vi "FTW-ActorTemplate.vi"(0 "FTW Actor Instance Configuration":string="{\n  \"Identity\": \"ActorName\",\n  \"InboxAddress\": \"inproc://*\",\n  \"LoggerAddress\": \"\",\n  \"DebugEnableInboxLogging\": false,\n  \"DebugEnableJobLogging\": false,\n  \"LauncherAddress\": \"\"\n}", 11 "ErrorIn":errorcluster) -> (15 "Error":errorcluster)   [LabVIEW 2013]
uses:
  source/actor/Instance/FTW-ActorInstance.lvclass
  source/actor/Message/Base/FTW-Message.lvclass
  source/actor/Instance/FTW-ActorInstance.lvclass/FTW-ActorInstance.ctl
  source/actor/JobSequencer/FTW-SEQ-Current.vi
  source/actor/Message/Request/FTW-Message-IncomingRequest.lvclass
panel:
  # "Inputs"
  # "Outputs"
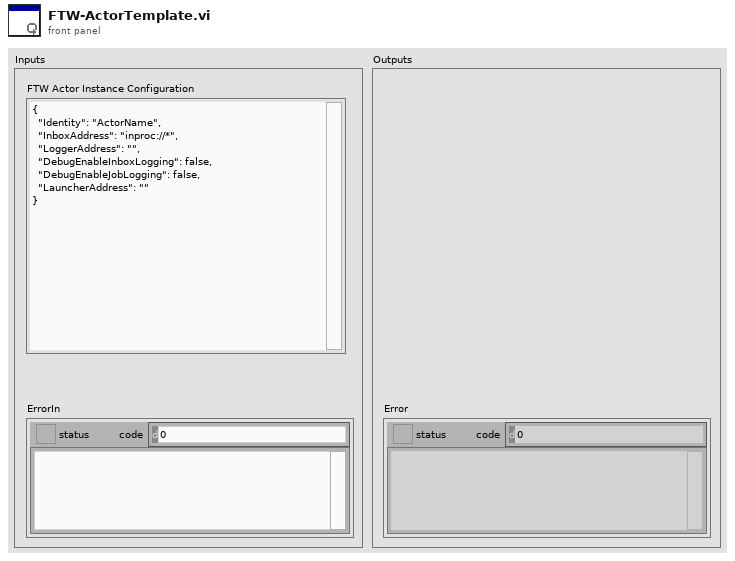
[diagram p1: front panel]
types:
  T1 = cluster{"Incoming Requests":refnum<event-registration>, "Local Messages":refnum<event-registration>, "Additional Registration Types":refnum<event-registration>}
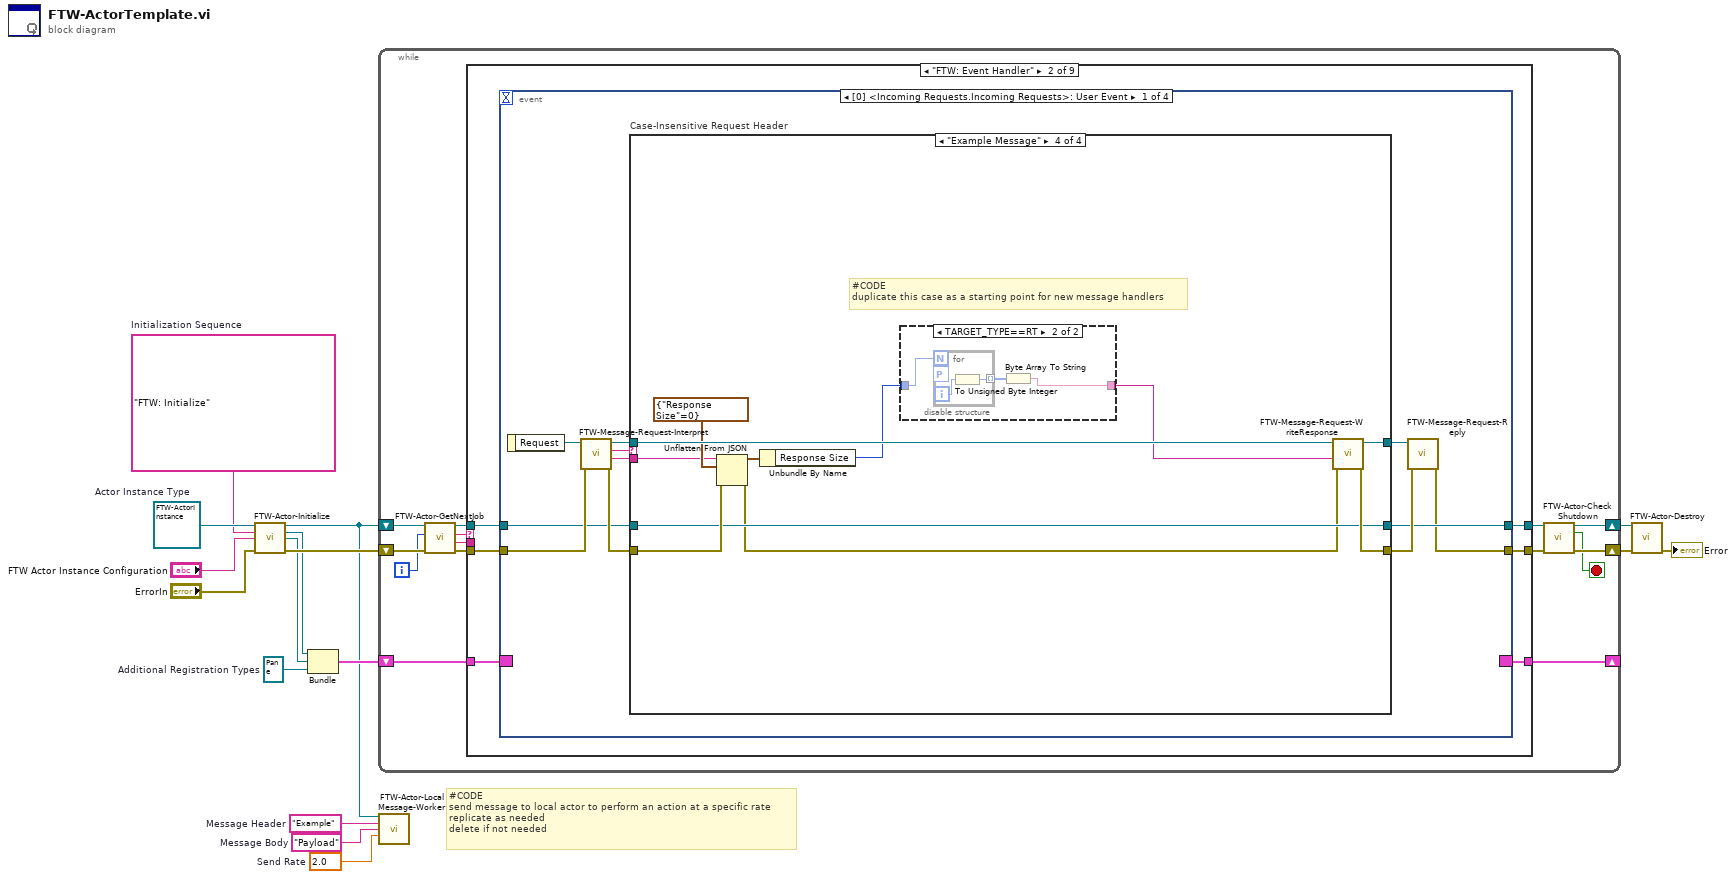
[diagram p0: block diagram]
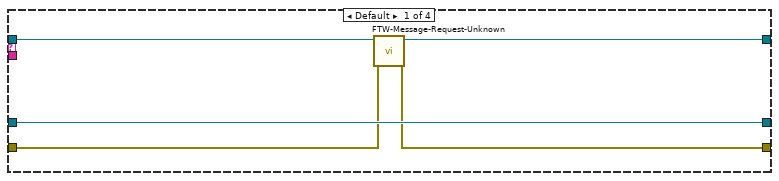
[diagram p3: hidden frame]
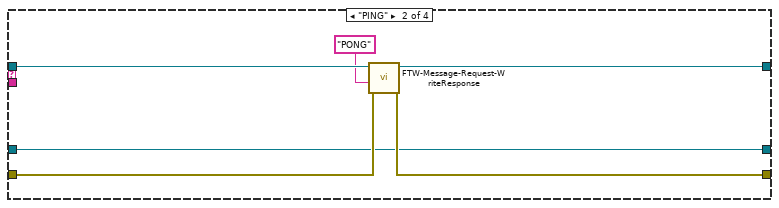
[diagram p4: hidden frame]
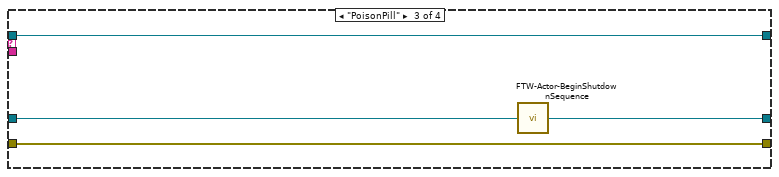
[diagram p5: hidden frame]
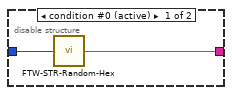
[diagram p6: hidden frame]
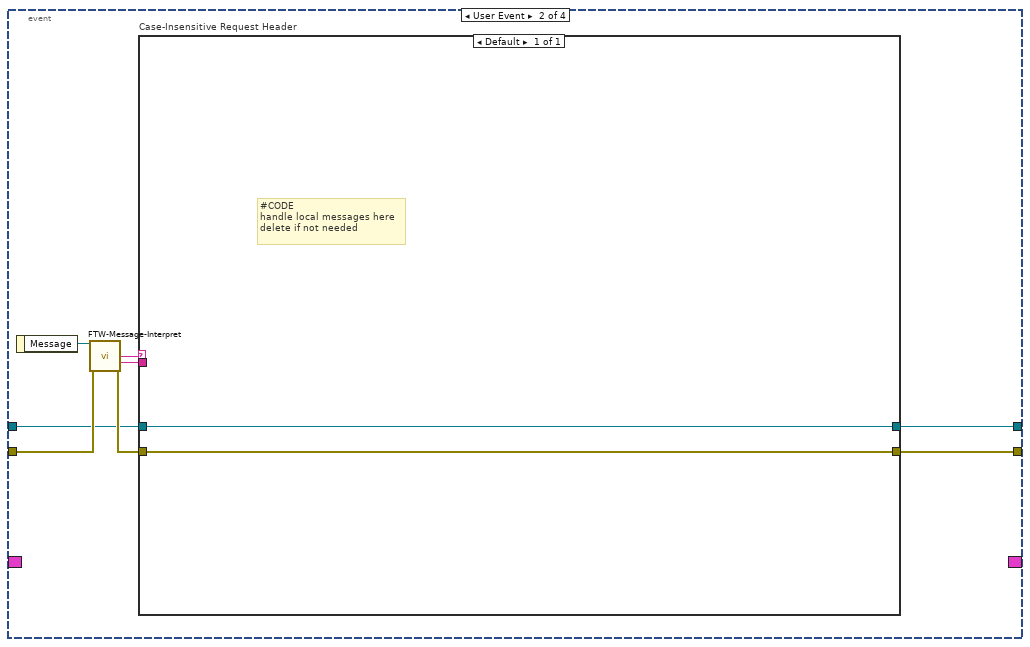
[diagram p7: hidden frame]
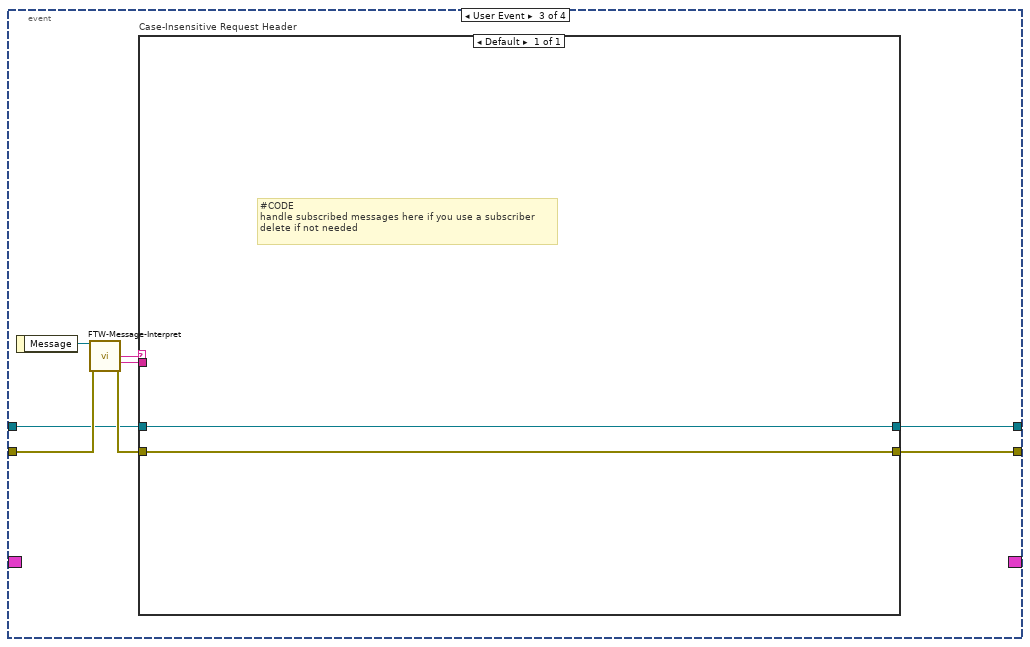
[diagram p8: hidden frame]
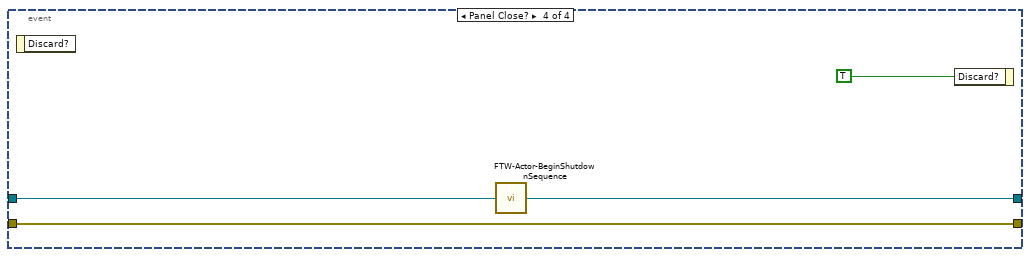
[diagram p9: hidden frame]
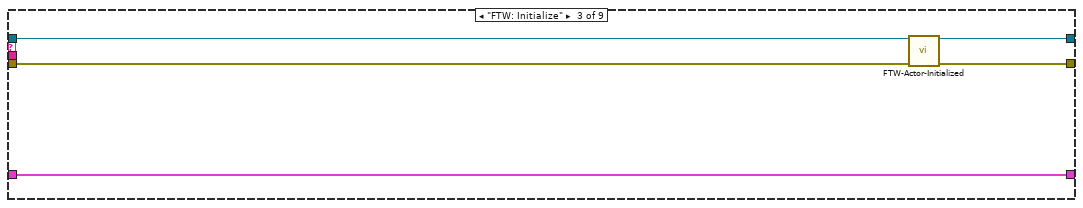
[diagram p10: hidden frame]
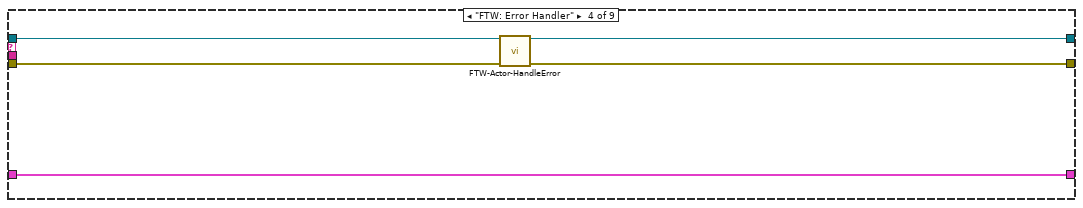
[diagram p11: hidden frame]
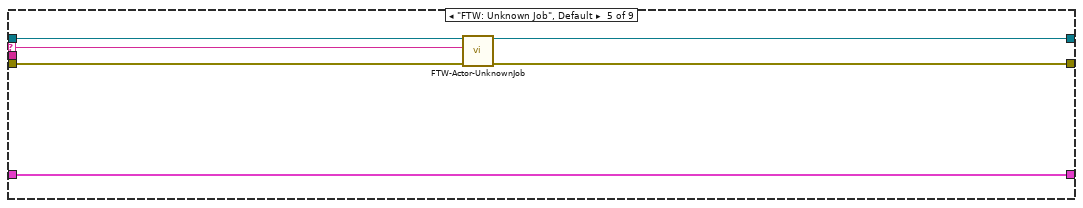
[diagram p12: hidden frame]
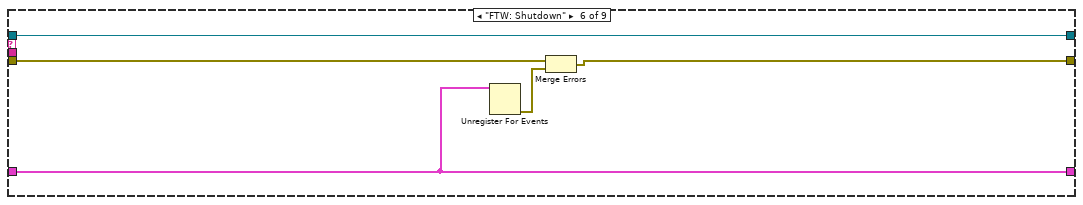
[diagram p13: hidden frame]
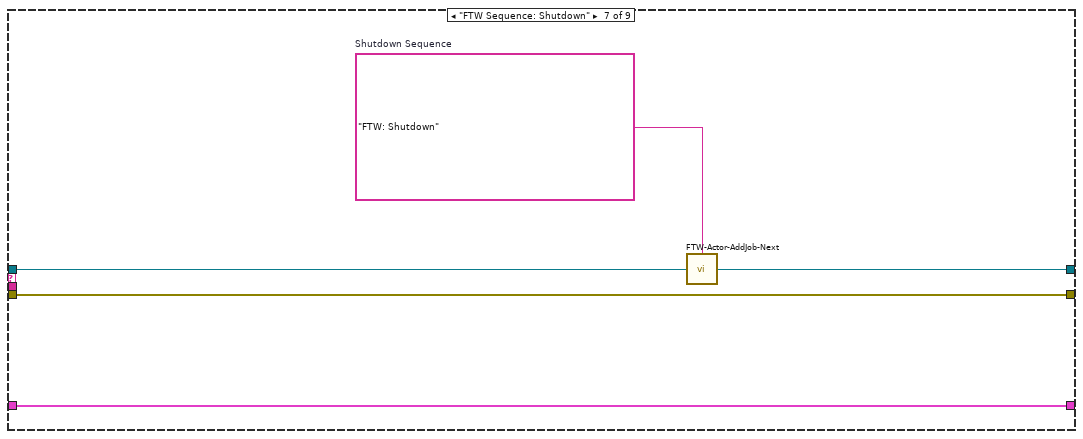
[diagram p14: hidden frame]
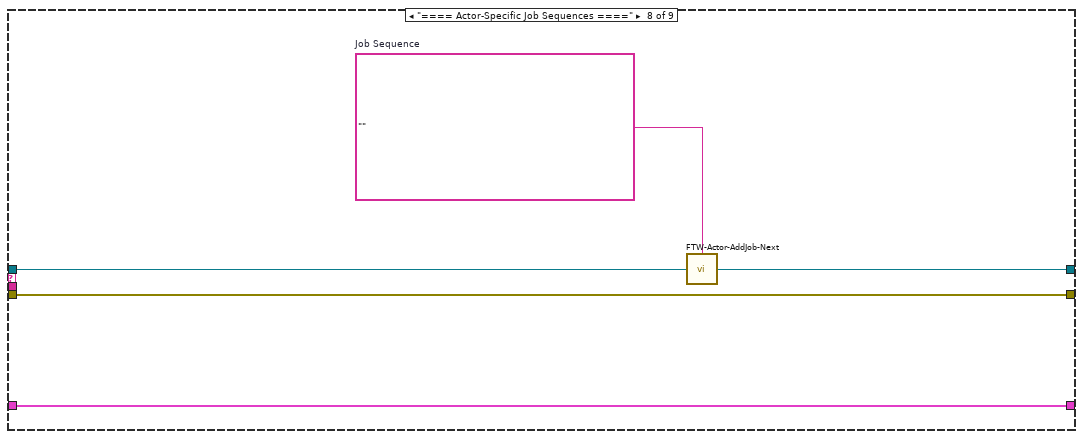
[diagram p15: hidden frame]
diagram:
  w1 = 2.0  # Send Rate
  w2 = "Payload"  # Message Body
  w3 = "Example"  # Message Header
  w5 = refnum<event-registration> refnum  # Additional Registration Types
  w12 = refnum<class "FTW-ActorInstance.lvclass"> refnum  # Actor Instance Type
  w11 = "FTW: Initialize"  # Initialization Sequence
  # "#CODE\nsend message to local actor to perform an action at a specific rate\nreplicate as needed\ndelete if not needed"
  n1 = call-dynamic "FTW-Actor-Initialize.vi"("FTW Actor Instance Type"=w12, "Initialization Job Sequence"=w11, "Actor Instance Configuration"="FTW Actor Instance Configuration", "error in"="ErrorIn") -> ("FTW Actor Instance"=w4:refnum<class "FTW-ActorInstance.lvclass">, "Incoming Requests"=w7:refnum<event-registration>, "Local Messages"=w6:refnum<event-registration>, "error out"=w13:errorcluster)  [unwired: 8 in]
  n2 = Bundle("Incoming Requests"=w7, "Local Messages"=w6, "Additional Registration Types"=w5) -> (w9:T1)  [unwired: 1 in]
  n3 = while {
    shift-right: [w20] -> w15
    shift-left: w13 -> [w27]
    shift-right: [w17] -> _
    shift-left: w9 -> [w30]
    shift-right: [w22] -> w16
    shift-left: w4 -> [w29]
    i -> [w18]
    stop <- w19 stop-if-true
    n4 = call "FTW-Actor-GetNextJob.vi"("error in"=w27, "Jobs Performed"=w18, "FTW Actor Instance"=w29) -> ("error out"=w26:errorcluster, "Job Data"=w24:string, "Job Name"=w25:string, "FTW Actor Instance out"=w28:refnum<class "FTW-ActorInstance.lvclass">)  [unwired: 5 in]
    n5 = case shown="\"FTW: Event Handler\"" w25 {
      selector: w25 -> [_ _ _ _ w118 _ _ _ _]
      tunnel: [w32 w39 w108 w113 w121 w127 w132 w137 w141] -> w21
      tunnel: w26 -> [w32 w38 w111 w115 w122 w128 w132 w137 w141]
      tunnel: w30 -> [w33 w34 w112 w117 w123 w124 w133 w138 w140]
      tunnel: [w33 w37 w112 w117 w123 w124 w133 w138 w140] -> w17
      tunnel: w24 -> [_ _ _ _ _ _ _ _ _]
      tunnel: [w31 w36 w109 w114 w119 w125 w130 w135 w139] -> w23
      tunnel: w28 -> [w31 w35 w110 w116 w120 w125 w131 w136 w139]
      frame "==== Featherweight Framework Jobs ====" {
      }
      frame "FTW: Event Handler" {
        n6 = event shown="[0] <Incoming Requests.Incoming Requests>: User Event" {
          selector: w34 -> [_ _ _ _]
          dyn-events: [_ _ _ _] -> w37
          timeout: _ -> [_ _ _ _]
          tunnel: [w42 w88 w98 w106] -> w39
          tunnel: w38 -> [w48 w89 w99 w106]
          tunnel: [w46 w87 w97 w104] -> w36
          tunnel: w35 -> [w45 w86 w96 w105]
          event User Event {
            n7 = event-data() -> ("Request"=w49:refnum<class "FTW-Message-IncomingRequest.lvclass">)  [unwired: 1 in]
            n8 = call "FTW-Message-Request-Interpret.vi"("error in"=w48, "FTW Incoming Request"=w49) -> ("error out"=w50:errorcluster, "Request Body"=w40:string, "Request Header"=w44:string, "FTW Incoming Request out"=w43:refnum<class "FTW-Message-IncomingRequest.lvclass">)  [unwired: 5 in, 1 out]
            n9 = case "Case-Insensitive Request Header" shown="\"Example Message\"" w44 {
              tunnel: [w53 w59 w64 w75] -> w47
              tunnel: w50 -> [w54 w60 w64 w76]
              tunnel: [w55 w58 w65 w72] -> w46
              tunnel: w45 -> [w55 w58 w63 w72]
              tunnel: w43 -> [w52 w61 w62 w74]
              tunnel: [w51 w57 w62 w73] -> w41
              tunnel: w40 -> [_ _ _ w66]
              frame Default {
                n10 = call "FTW-Message-Request-Unknown.vi"("error in"=w54, "FTW Incoming Request"=w52) -> ("error out"=w53:errorcluster, "FTW Incoming Request Out"=w51:refnum<class "FTW-Message-IncomingRequest.lvclass">)  [unwired: 8 in]
              }
              frame "PING" {
                n11 = call "FTW-Message-Request-WriteResponse.vi"("error in"=w60, "Response Body"="PONG" ("Response Header"), "FTW Incoming Request"=w61) -> ("error out"=w59:errorcluster, "FTW Incoming Request out"=w57:refnum<class "FTW-Message-IncomingRequest.lvclass">)  [unwired: 7 in]
              }
              frame "PoisonPill" {
                n12 = call "FTW-Actor-BeginShutdownSequence.vi"("FTW Actor Instance"=w63) -> ("FTW Actor Instance out"=w65:refnum<class "FTW-ActorInstance.lvclass">)  [unwired: 3 in]
              }
              frame "Example Message" {
                # "#CODE\nduplicate this case as a starting point for new message handlers"
                n13 = Unflatten From JSON(JSON string=w66, type and defaults=cluster{"Response Size":i32} {"Response Size"=0}, error in (no error)=w76) -> (value=w69:cluster{"Response Size":i32}, error out=w71:errorcluster)  [unwired: 4 in]
                n14 = Unbundle By Name(w69) -> ("Response Size"=w68:i32)
                n15 = disable-structure shown="TARGET_TYPE==RT" {
                  disable-tunnel: w68 -> [w78 w81]
                  disable-tunnel: [w77 w79] -> w67
                  frame condition #0 (active) {
                    n16 = call "FTW-STR-Random-Hex.vi"("String Length"=w78) -> ("Random Hex String"=w77:string)  [unwired: 3 in]
                  }
                  frame condition #1 {
                    n17 = for {
                      N: w81 -> [_]
                      workers-P: _ -> [_]
                      tunnel: [w82] -> w80 mode=indexing
                      i -> [w83]
                      n18 = To Unsigned Byte Integer(number=w83) -> (unsigned 8bit integer=w82:u8)
                    }
                    n19 = Byte Array To String(unsigned byte array=w80) -> (string=w79:string)
                  }
                }
                n20 = call "FTW-Message-Request-WriteResponse.vi"("error in"=w71, "Response Body"=w67, "FTW Incoming Request"=w74) -> ("error out"=w75:errorcluster, "FTW Incoming Request out"=w73:refnum<class "FTW-Message-IncomingRequest.lvclass">)  [unwired: 7 in]
              }
            }
            n21 = call "FTW-Message-Request-Reply.vi"("FTW: Reply Error"=w47, "FTW Incoming Request"=w41) -> ("error out"=w42:errorcluster)  [unwired: 8 in, 1 out]
          }
          event User Event {
            n22 = event-data() -> ("Message"=w90:refnum<class "FTW-Message.lvclass">)  [unwired: 1 in]
            n23 = call-dynamic "FTW-Message-Interpret.vi"("FTW Message"=w90, "error in"=w89) -> ("Message Header"=w84:string, "Message Body"=w85:string, "error out"=w91:errorcluster)  [unwired: 9 in, 2 out]
            n24 = case "Case-Insensitive Request Header" shown="Default" w84 {
              tunnel: [w92] -> w88
              tunnel: w91 -> [w92]
              tunnel: [w93] -> w87
              tunnel: w86 -> [w93]
              tunnel: w85 -> [_]
              frame Default {
                # "#CODE\nhandle local messages here\ndelete if not needed"
              }
            }
          }
          event User Event {
            n25 = event-data() -> ("Message"=w100:refnum<class "FTW-Message.lvclass">)  [unwired: 1 in]
            n26 = call-dynamic "FTW-Message-Interpret.vi"("FTW Message"=w100, "error in"=w99) -> ("Message Header"=w94:string, "Message Body"=w95:string, "error out"=w101:errorcluster)  [unwired: 9 in, 2 out]
            n27 = case "Case-Insensitive Request Header" shown="Default" w94 {
              tunnel: [w102] -> w98
              tunnel: w101 -> [w102]
              tunnel: [w103] -> w97
              tunnel: w96 -> [w103]
              tunnel: w95 -> [_]
              frame Default {
                # "#CODE\nhandle subscribed messages here if you use a subscriber\ndelete if not needed"
              }
            }
          }
          event Panel Close? {
            n28 = event-data() -> ()  [unwired: 1 in, 1 out]
            n29 = call "FTW-Actor-BeginShutdownSequence.vi"("FTW Actor Instance"=w105) -> ("FTW Actor Instance out"=w104:refnum<class "FTW-ActorInstance.lvclass">)  [unwired: 3 in]
            n30 = event-data("Discard?"=TRUE) -> ()  [unwired: 1 in, 1 out]
          }
        }
      }
      frame "FTW: Initialize" {
        n31 = call-dynamic "FTW-Actor-Initialized.vi"("FTW Actor Instance"=w110, "error in"=w111) -> ("FTW Actor Instance out"=w109:refnum<class "FTW-ActorInstance.lvclass">, "error out"=w108:errorcluster)  [unwired: 12 in]
      }
      frame "FTW: Error Handler" {
        n32 = call-dynamic "FTW-Actor-HandleError.vi"("FTW Actor Instance"=w116, "error in"=w115) -> ("FTW Actor Instance out"=w114:refnum<class "FTW-ActorInstance.lvclass">, "error out"=w113:errorcluster)  [unwired: 11 in, 1 out]
      }
      frame "FTW: Unknown Job", Default {
        n33 = call-dynamic "FTW-Actor-UnknownJob.vi"("FTW Actor Instance"=w120, "Unknown Job"=w118, "error in"=w122) -> ("FTW Actor Instance out"=w119:refnum<class "FTW-ActorInstance.lvclass">, "error out"=w121:errorcluster)  [unwired: 11 in]
      }
      frame "FTW: Shutdown" {
        n34 = Unregister For Events(event registration refnum=w124) -> (error out=w126:errorcluster)  [unwired: 1 in]
        n35 = Merge Errors(w128, w126) -> (w127:errorcluster)
      }
      frame "FTW Sequence: Shutdown" {
        w129 = "FTW: Shutdown"  # Shutdown Sequence
        n36 = call "FTW-Actor-AddJob-Next.vi"("Add Next in Job Queue"=w129, "FTW Actor Instance"=w131) -> ("FTW Actor Instance out"=w130:refnum<class "FTW-ActorInstance.lvclass">)  [unwired: 2 in]
      }
      frame "==== Actor-Specific Job Sequences ====" {
        w134 = ""  # Job Sequence
        n37 = call "FTW-Actor-AddJob-Next.vi"("Add Next in Job Queue"=w134, "FTW Actor Instance"=w136) -> ("FTW Actor Instance out"=w135:refnum<class "FTW-ActorInstance.lvclass">)  [unwired: 2 in]
      }
      frame "==== Actor-Specific Jobs ====" {
      }
    }
    n38 = call "FTW-Actor-CheckShutdown.vi"("FTW Actor Instance"=w23, "error in"=w21) -> ("FTW Actor Instance out"=w22:refnum<class "FTW-ActorInstance.lvclass">, "Shutdown?"=w19:bool, "error out"=w20:errorcluster)  [unwired: 11 in]
  }
  n39 = call-dynamic "FTW-Actor-LocalMessage-Worker.vi"("FTW-ActorInstance In"=w4, "Message Header"=w3, "Message Body"=w2, "Send Rate"=w1) -> ()  [unwired: 11 in, 1 out]
  n40 = call-dynamic "FTW-Actor-Destroy.vi"("FTW Actor Instance"=w16, "error in"=w15) -> ("error out"=→"Error":errorcluster)  [unwired: 13 in]
